vi "Digital Input.vi"() -> ()   [LabVIEW 2009]
uses:
  <vilib>/DAQmx/create/channels.llb/DAQmx Create Channel (DI-Digital Input).vi
  <vilib>/DAQmx/read.llb/DAQmx Read (Digital Bool 1Line 1Point).vi
  Program Files (x86)/National Instruments/LabVIEW 2009/resource/objmgr/daqmx.rc
panel:
  in  "stop":bool
  out "data":bool
  in  "lines":tag
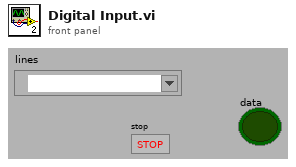
[diagram p1: front panel]
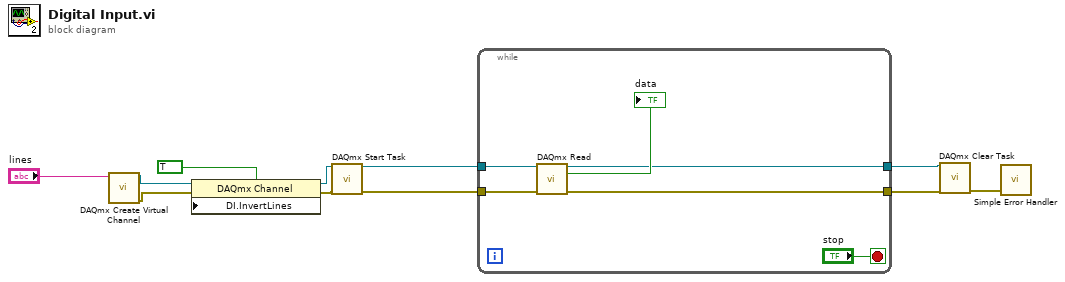
[diagram p0: block diagram]
diagram:
  n1 = call-poly <vilib>:"DAQmx Create Virtual Channel.vi"("lines"="lines") -> ("task out"=w4:refnum<k21>, "error out"=w3:errorcluster)  [unwired: 13 in]
  n2 = property class="DAQmx Channel"(reference=w4, error in=w3, "DI.InvertLines"=TRUE) -> (reference out=w5:refnum<k21>, error out=w2:errorcluster)
  n3 = call <vilib>:"DAQmx Start Task.vi"("task/channels in"=w5, "error in"=w2) -> ("task out"=w10:refnum<k21>, "error out"=w9:errorcluster)  [unwired: 12 in]
  n4 = while {
    tunnel: w10 -> [w17]
    tunnel: w9 -> [w16]
    tunnel: [w13] -> w8
    tunnel: [w12] -> w7
    stop <- "stop" stop-if-true
    n5 = call-poly <vilib>:"DAQmx Read.vi"("task/channels in"=w17, "error in"=w16) -> ("task out"=w13:refnum<k21>, "data"=→"data":bool, "error out"=w12:errorcluster)  [unwired: 11 in]
  }
  n6 = call <vilib>:"DAQmx Clear Task.vi"("task in"=w8, "error in"=w7) -> ("error out"=w6:errorcluster)  [unwired: 13 in]
  n7 = call <vilib>:"Simple Error Handler.vi"("error in (no error)"=w6) -> ()  [unwired: 4 in, 5 out]
